vi "Auto Unload Callback.vi"(4 "Sequence Context":T2) -> (0 "error out":errorcluster, 1 "Test Data":T1 {"Numeric Measurement" format="%.2f"})   [LabVIEW 2011]
uses:
  <vilib>/addons/TestStand/_TSLegacy.llb/LabVIEW Test - Sequence Context.ctl
  <vilib>/addons/TestStand/_TSLegacy.llb/LabVIEW Test - Test Data.ctl
panel:
  in  "Accept":bool
  in  "Power Switch":bool
  # "Power must be off\nbefore unloading sequence"
  # "On"
  # "Off"
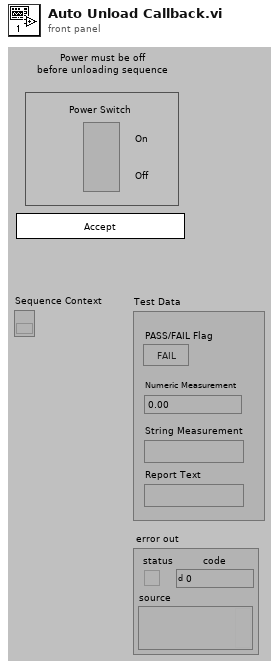
[diagram p1: front panel]
types:
  T1 = typedef "LabVIEW Test - Test Data.ctl" = cluster{"PASS/FAIL Flag":bool, "Numeric Measurement":dbl, "String Measurement":string, "Report Text":string}
  T2 = typedef "LabVIEW Test - Sequence Context.ctl" = refnum<k7>
  T3 = typedef "TestStand - Status Monitor.ctl" = cluster{"Sequence Context":refnum<k7>, "Execution":refnum<k7>, "Termination Monitor":refnum<k7>}
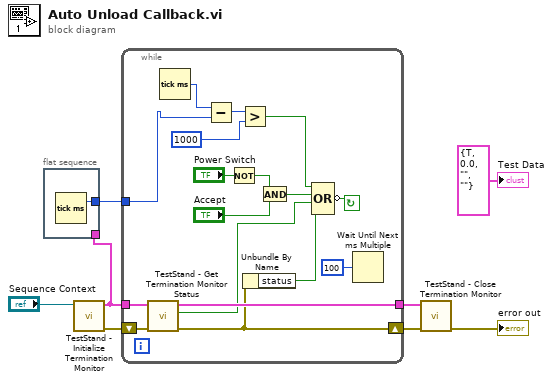
[diagram p0: block diagram]
diagram:
  n1 = flat-sequence {
    tunnel: [w9] -> w1
    tunnel: w2 -> [_]
    frame #0 {
      n2 = Tick Count (ms)() -> (millisecond timer value=w9:u32)
    }
  }
  n3 = call <vilib>:"TestStand - Initialize Termination Monitor.vi"("Sequence Context In"="Sequence Context") -> ("error out"=w7:errorcluster, "Status Monitor Out"=w2:T3)  [unwired: 1 in, 8 out]
  n4 = while {
    tunnel: [w18] -> w3
    tunnel: w2 -> [w19]
    shift-left: w7 -> [w20]
    shift-right: [w17] -> w6
    tunnel: w1 -> [w11]
    stop <- w23 continue-if-true
    n5 = call <vilib>:"TestStand - Get Termination Monitor Status.vi"("error in (no error)"=w20, "Status Monitor In"=w19) -> ("error out"=w17:errorcluster, "Terminating or Aborting"=w16:bool, "Status Monitor Out"=w18:T3)  [unwired: 7 out]
    n6 = Tick Count (ms)() -> (millisecond timer value=w13:u32)
    n7 = Subtract(x=w13, y=w11) -> (x-y=w14:u32)
    n8 = Not(x="Power Switch") -> (.not. x?=w21:bool)
    n9 = Greater?(x=w14, y=u32 1000) -> (0:w10:bool)
    n10 = Unbundle By Name(w17) -> ("status"=w15:bool)
    n11 = And(x=w21, y="Accept") -> (x .and. y?=w24:bool)
    n12 = Compound Arithmetic op=OR(w10, w24, w16, w15) -> (invert w23:bool)
    n13 = Wait Until Next ms Multiple(millisecond multiple=u32 100) -> ()  [unwired: 1 out]
  }
  n14 = call <vilib>:"TestStand - Close Termination Monitor.vi"("error in (no error)"=w6, "Status Monitor In"=w3) -> ("error out"=→"error out":errorcluster)  [unwired: 9 out]
  "Test Data" <- T1 {"PASS/FAIL Flag"=TRUE, "Numeric Measurement"=0.0, "String Measurement"="", "Report Text"=""} ("Test Data")
